vi "galvo_triangle_wave.vi"(8 "trial seconds":dbl=1.0, 9 "final frequency":dbl, 10 "amplitude":dbl=1.0 format="%0.2f", 11 "sample rate":dbl) -> (2 "waveform array out":waveform(dbl)[](array[waveform]))   [LabVIEW 2025]
uses:
  <vilib>/Analysis/NI_AALBase.lvlib
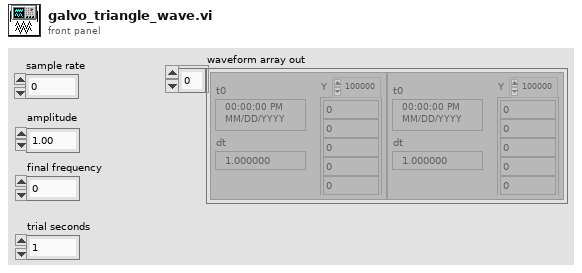
[diagram p1: front panel]
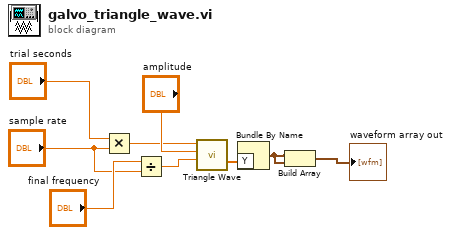
[diagram p0: block diagram]
diagram:
  n1 = Multiply(x="trial seconds", y="sample rate") -> (x*y=w4:dbl)
  n2 = Divide(x="final frequency", y="sample rate") -> (x/y=w9:dbl)
  n3 = call <vilib>:"Triangle Wave.vi"("samples"=w4, "amplitude"="amplitude", "frequency"=w9) -> ("triangle wave"=w8:dbl[])  [unwired: 2 in, 2 out]
  n4 = Bundle By Name("Y"=w8) -> (w6:waveform(dbl))  [unwired: 1 in]
  n5 = Build Array(w6, w6) -> (→"waveform array out":waveform(dbl)[])
